vi "Create myQuake.vi"(8 "error in (no error)":errorcluster, 9 "rate (500 Hz)":dbl=500.0, 10 "device name (myDAQ1)":tag="myDAQ1") -> (0 "error out":errorcluster, 2 "connection failed?":bool, 3 "task array out":refnum<k21>[](array[refnum]))   [LabVIEW 2013]
doc: "Creates an array of 3 DAQmx tasks used in myQuake\n\nUse the <b> device name</b> input to select the preferred device. The first available myDAQ will be used if the preferred device is not found.\nThe <b>rate</b> sets the acquisition rate on the accelerometer channels.\n\nAnalog Input 0:1 Accelerometer A and B\nAnalog Output 0 Quake Motor Drive\nDigital Outputs\n D0:1 A MUX Control\n D2 A Sensitivity\n D4:5 B MUX Control\n D6 B Sensitivity\n D7 Accelerometer Power (Always On)\n (D3 not used in task)"
uses:
  <vilib>/DAQmx/create/channels.llb/DAQmx Create Channel (AI-Voltage-Basic).vi
  <vilib>/DAQmx/configure/timing.llb/DAQmx Timing (Sample Clock).vi
  <vilib>/DAQmx/create/channels.llb/DAQmx Create Channel (AO-Voltage-Basic).vi
  <vilib>/DAQmx/create/channels.llb/DAQmx Create Channel (DO-Digital Output).vi
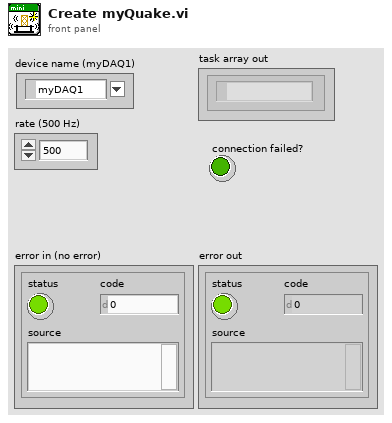
[diagram p1: front panel]
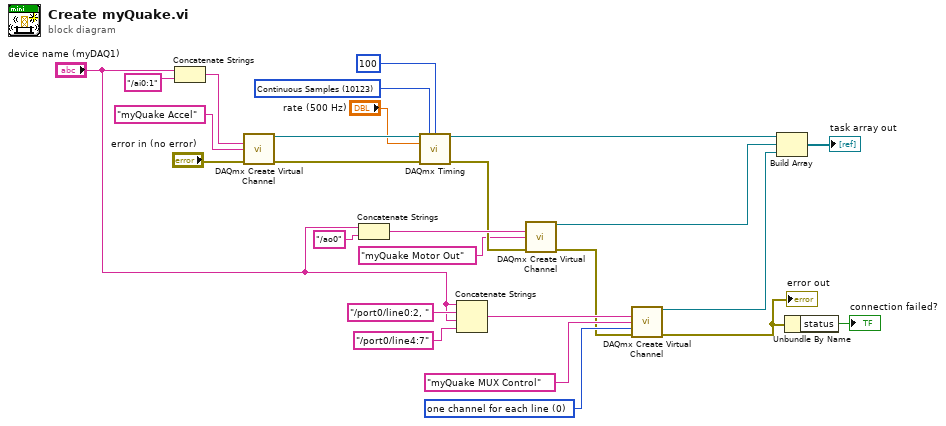
[diagram p0: block diagram]
diagram:
  w14 = 10123 items=["Finite Samples"=10178, "Continuous Samples"=10123, "Hardware Timed Single Point"=12522] ("sample mode")
  w19 = 0 items=["one channel for each line", "one channel for all lines"] ("line grouping")
  n1 = Concatenate Strings("device name (myDAQ1)", "/ai0:1" ("string")) -> (w21:string)
  n2 = call-poly <vilib>:"DAQmx Create Virtual Channel.vi"("physical channels"=w21, "name to assign"="myQuake Accel" ("Descr (myDAQ AI)"), "error in"="error in (no error)") -> ("task out"=w9:refnum<k21>, "error out"=w15:errorcluster)  [unwired: 11 in]
  n3 = Concatenate Strings("device name (myDAQ1)", "/ao0" ("string")) -> (w20:string)
  n4 = call-poly <vilib>:"DAQmx Timing.vi"("task/channels in"=w9, "sample mode"=w14, "samples per channel"=100, "rate"="rate (500 Hz)", "error in"=w15) -> ("task out"=w10:refnum<k21>, "error out"=w12:errorcluster)  [unwired: 9 in]
  n5 = Concatenate Strings("device name (myDAQ1)", "/port0/line0:2, " ("string"), "device name (myDAQ1)", "/port0/line4:7" ("string")) -> (w18:string)
  n6 = call-poly <vilib>:"DAQmx Create Virtual Channel.vi"("physical channels"=w20, "name to assign"="myQuake Motor Out", "error in"=w12) -> ("task out"=w8:refnum<k21>, "error out"=w11:errorcluster)  [unwired: 11 in]
  n7 = call-poly <vilib>:"DAQmx Create Virtual Channel.vi"("lines"=w18, "name to assign"="myQuake MUX Control" ("Channel Description"), "line grouping"=w19, "error in"=w11) -> ("task out"=w7:refnum<k21>, "error out"=w1:errorcluster)  [unwired: 10 in]
  "error out" <- w1
  n8 = Build Array(w10, w8, w7) -> (→"task array out":refnum<k21>[])
  n9 = Unbundle By Name(w1) -> ("status"=→"connection failed?":bool)
